vi "Read MethodRefnum.vi"(8 "error in (no error)":errorcluster, 11 "CS++Methods in":refnum<class "CS++Method.lvclass">) -> (0 "error out":errorcluster, 2 "MethodRefnum":refnum<vi>, 3 "CS++Methods out":refnum<class "CS++Method.lvclass">)   [LabVIEW 2015, in "CS++Method.lvlib" / "CS++Method.lvclass"]
uses:
  CS++Method.lvclass
  CS++Method.lvclass/CS++Method.ctl
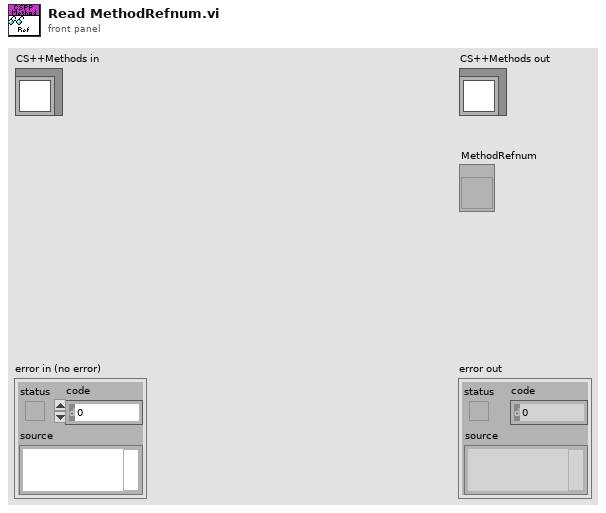
[diagram p1: front panel]
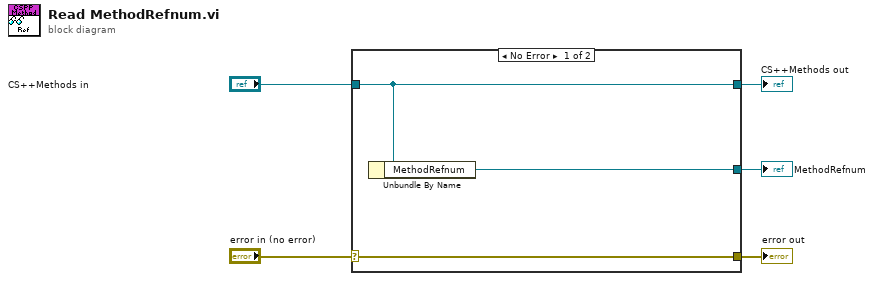
[diagram p0: block diagram]
diagram:
  n1 = case shown="No Error" "error in (no error)" {
    selector: "error in (no error)" -> [w8 w9]
    tunnel: [w8 w9] -> w4
    tunnel: [w7 w10] -> w2
    tunnel: "CS++Methods in" -> [w7 w10]
    tunnel: [w6 _] -> w1
    frame No Error {
      n2 = Unbundle By Name(w7) -> ("MethodRefnum"=w6:refnum<vi>)
    }
    frame Error {
    }
  }
  "error out" <- w4
  "CS++Methods out" <- w2
  "MethodRefnum" <- w1
